vi "disable_compression.vi"(7 "connection_reference":T1, 8 "error in (no error)":errorcluster, 11 "hyper_table_name":string) -> (0 "error out":errorcluster)   [LabVIEW 2015, in "lv-timescaledb.lvlib"]
uses:
  lv-timescaledb.lvlib
  <vilib>/addons/database/Connection.llb/Conn ObjectReference.ctl
  <vilib>/addons/database/Command.llb/Cmd Execute.vi
  <vilib>/addons/database/Recordset.llb/Rec Destroy - Command.vi
  <vilib>/addons/database/Command.llb/Cmd Delete.vi
  <vilib>/addons/database/NI_Database_API.lvlib
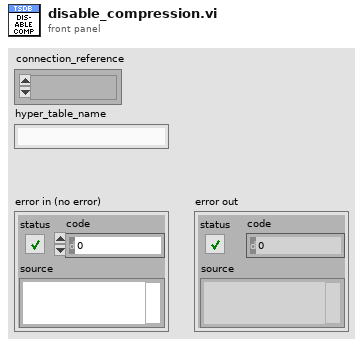
[diagram p1: front panel]
types:
  T1 = typedef "NI_Database_API.lvlib/Conn ObjectReference.ctl" = refnum<k1>
  T2 = typedef "NI_Database_API.lvlib/Cmd ObjectReference.ctl" = refnum<k1>
  T3 = typedef "NI_Database_API.lvlib/Cmd-Rec Object Reference.ctl" = refnum<k1>
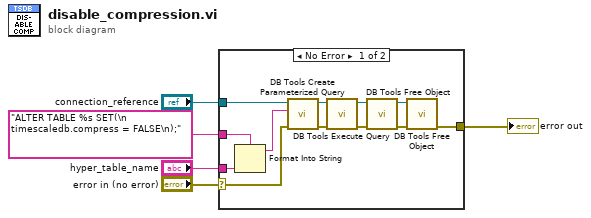
[diagram p0: block diagram]
diagram:
  n1 = case shown="No Error" "error in (no error)" {
    selector: "error in (no error)" -> [w7 w18]
    tunnel: "hyper_table_name" -> [w6 _]
    tunnel: "connection_reference" -> [w17 _]
    tunnel: [w16 w18] -> w3
    tunnel: "ALTER TABLE %s SET(\n    timescaledb.compress = FALSE\n);" -> [w9 _]
    frame No Error {
      n2 = Format Into String(format string=w9, w6) -> (resulting string=w8:string)  [unwired: 2 in, 1 out]
      n3 = call <vilib>:"DB Tools Create Parameterized Query.vi"("error in (no error)"=w7, "SQL query"=w8, "connection reference"=w17) -> ("error out"=w14:errorcluster, "command reference"=w12:T2)  [unwired: 4 in, 1 out]
      n4 = call-poly <vilib>:"DB Tools Execute Query.vi"("error in (no error)"=w14, "command reference"=w12) -> ("error out"=w15:errorcluster, "command-recordset reference"=w11:T3)  [unwired: 6 in]
      n5 = call-poly <vilib>:"DB Tools Free Object.vi"("error in (no error)"=w15, "command-recordset reference"=w11) -> ("error out"=w13:errorcluster, "command reference"=w10:T2)  [unwired: 8 in]
      n6 = call-poly <vilib>:"DB Tools Free Object.vi"("error in (no error)"=w13, "command reference"=w10) -> ("error out"=w16:errorcluster)  [unwired: 8 in, 1 out]
    }
    frame Error {
    }
  }
  "error out" <- w3
